vi "Write_Safe.vi"(3 "error in":errorcluster, 4 "Data":string, 5 "refnum":refnum<file>) -> (0 "error out":errorcluster, 1 "Explorer Launch error":i32, 2 "dup refnum":refnum<file>)   [LabVIEW 2017]
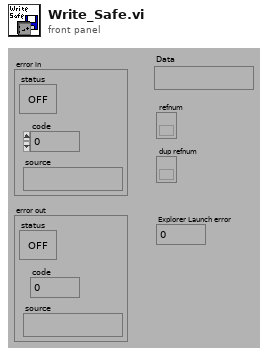
[diagram p1: front panel]
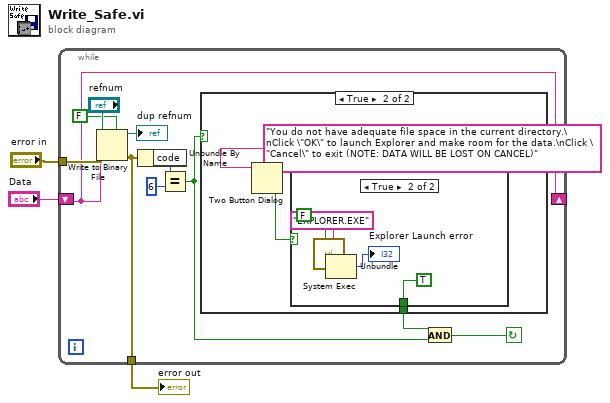
[diagram p0: block diagram]
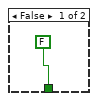
[diagram p2: hidden frame]
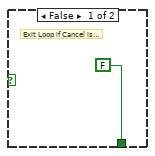
[diagram p3: hidden frame]
diagram:
  n1 = while {
    shift-left: "Data" -> [w8]
    shift-right: [w8] -> _
    tunnel: [w13] -> w2
    tunnel: "error in" -> [w14]
    stop <- w5 continue-if-true
    n2 = Write to Binary File(file (use dialog)="refnum", data=w8, error in=w14, 5:FALSE ("prepend array or string size? (T)")) -> (refnum out=→"dup refnum":refnum<file>, error out=w13:errorcluster)  [unwired: 2 in, 1 out]
    n3 = Unbundle By Name(w13) -> ("code"=w12:i32)
    n4 = Equal?(x=w12, y=6) -> (x = y?=w6:bool)
    n5 = case shown="True" w6 {
      tunnel: [FALSE w16] -> w7
      frame False {
      }
      frame True {
        n6 = Two Button Dialog(message="You do not have adequate file space in the current directory.\nClick \"OK\" to launch Explorer and make room for the data.\nClick \"Cancel\" to exit (NOTE: DATA WILL BE LOST ON CANCEL)") -> (T button?=w17:bool)  [unwired: 2 in]
        n7 = case shown="True" w17 {
          tunnel: [FALSE TRUE] -> w16
          frame False {
            # "Exit Loop if Cancel is selected"
          }
          frame True {
            n8 = call <vilib>:"System Exec.vi"("wait until completion? (T)"=FALSE, "command line"="EXPLORER.EXE" ("command to execute")) -> ("error out"=w21:errorcluster)  [unwired: 6 in, 3 out]
            n9 = Unbundle(w21) -> ("code"=→"Explorer Launch error":i32)  [unwired: 2 out]
          }
        }
      }
    }
    n10 = And(x=w7, y=w6) -> (x .and. y?=w5:bool)
  }
  "error out" <- w2
